vi "LiftMain.vi"(8 "Error In":errorcluster, 9 "Down":bool, 10 "Up":bool, 11 "Mode":enum16{"Open", "Control"}(ring)) -> (0 "Error Out":errorcluster)   [LabVIEW 2017]
uses:
  <vilib>/Rock Robotics/SystemInterfaces/DIO/FPGA_DIORelayChannel.ctl
  <vilib>/Rock Robotics/WPI/Relay/WPI_RelayDirection.ctl
  <vilib>/Rock Robotics/WPI/Relay/WPI_RelayValue.ctl
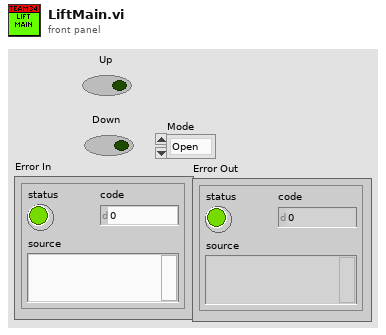
[diagram p1: front panel]
types:
  T1 = typedef "WPI_RelayDirection.ctl" = enum16{"Both directions", "Forward only", "Reverse only"}
  T2 = typedef "FPGA_DIORelayChannel.ctl" = enum8{"Relay 0", "Relay 1", "Relay 2", "Relay 3", "Invalid"}
  T3 = typedef "WPI_RelayValue.ctl" = enum16{"Off", "On", "Forward", "Reverse"}
  T4 = typedef "WPI_RelayDevRef.ctl" = cluster{"DevStatus":errorcluster, "Relay Channel":T2, "Relay Direction":T1}
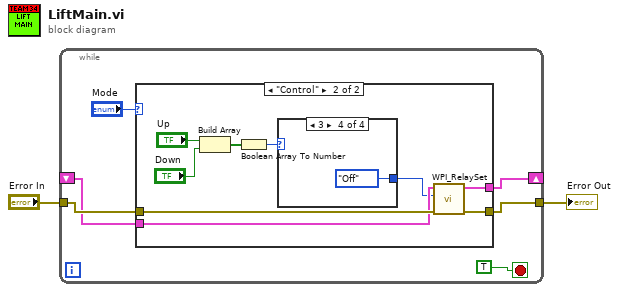
[diagram p0: block diagram]
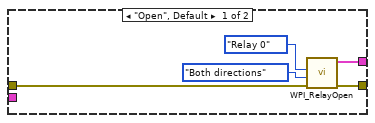
[diagram p2: hidden frame]
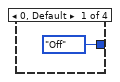
[diagram p3: hidden frame]
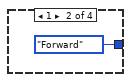
[diagram p4: hidden frame]
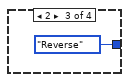
[diagram p5: hidden frame]
diagram:
  n1 = while {
    tunnel: "Error In" -> [w8]
    tunnel: [w7] -> w1
    shift-right: [w5] -> _
    shift-left: _ -> [w4]
    stop <- TRUE stop-if-true
    n2 = case shown="\"Control\"" "Mode" {
      tunnel: [w10 w21] -> w7
      tunnel: w8 -> [w11 w20]
      tunnel: [w13 w22] -> w5
      tunnel: w4 -> [_ w19]
      frame "Open", Default {
        n3 = call <vilib>:"WPI_RelayOpen.vi"("error in (no error)"=w11, "Relay Direction"=WPI_RelayDirection."Both directions", "Relay Channel"=FPGA_DIORelayChannel."Relay 0") -> ("error out"=w10:errorcluster, "RelayDevRef"=w13:T4)  [unwired: 7 in]
      }
      frame "Control" {
        n4 = Build Array("Up", "Down") -> (w16:bool[])
        n5 = Boolean Array To Number(Boolean array=w16) -> (number=w15:u32)
        n6 = case shown="3" w15 {
          tunnel: [WPI_RelayValue."Off" ("RelayValue") WPI_RelayValue."Forward" ("RelayValue") WPI_RelayValue."Reverse" ("RelayValue") WPI_RelayValue."Off" ("RelayValue")] -> w14
          frame 0, Default {
          }
          frame 1 {
          }
          frame 2 {
          }
          frame 3 {
          }
        }
        n7 = call <vilib>:"WPI_RelaySet.vi"("error in (no error)"=w20, "RelayValue"=w14, "RelayDevRef"=w19) -> ("error out"=w21:errorcluster, "RelayDevRef"=w22:T4)  [unwired: 7 in]
      }
    }
  }
  "Error Out" <- w1
